vi "Open Method Front Panel.vi"(8 "error in (no error)":errorcluster, 10 "String":string, 11 "Execution UI In":refnum<class "Execution UI.lvclass">) -> (0 "error out":errorcluster, 3 "Execution UI Out":refnum<class "Execution UI.lvclass">)   [LabVIEW 2020, in "Execution UI.lvclass"]
uses:
  Execution UI.lvclass
  Execution UI.lvclass/Execution UI.ctl
  Helper Classes/Test Finder/Test Finder.lvclass
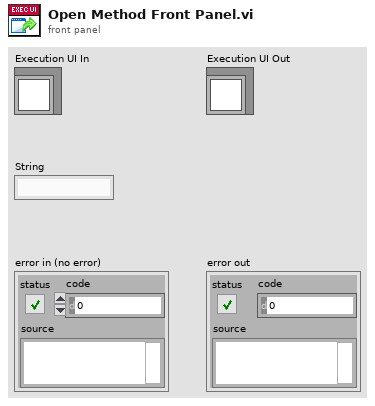
[diagram p1: front panel]
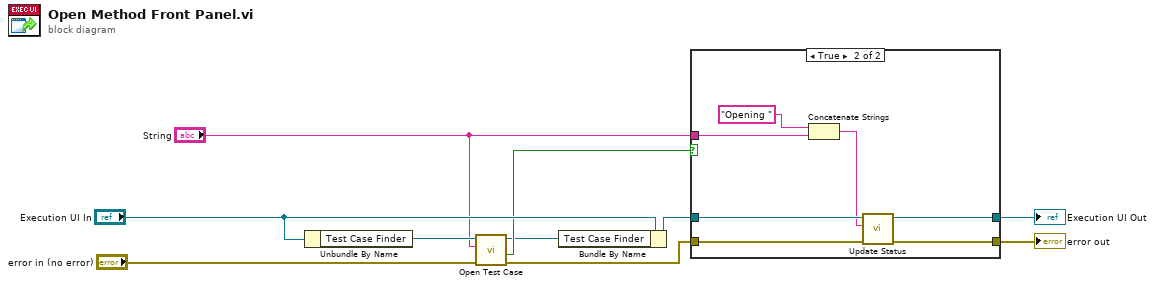
[diagram p0: block diagram]
diagram:
  n1 = Unbundle By Name("Execution UI In") -> ("Test Case Finder"=w10:refnum<class "Test Finder.lvclass">)
  n2 = call-dynamic "Open Test Case.vi"("error in (no error)"="error in (no error)", "Tag"="String", "Test Finder In"=w10) -> ("error out"=w6:errorcluster, "VI name valid?"=w7:bool, "Test Finder Out"=w1:refnum<class "Test Finder.lvclass">)  [unwired: 6 in]
  n3 = Bundle By Name(cluster="Execution UI In", "Test Case Finder"=w1) -> (w2:refnum<class "Execution UI.lvclass">)
  n4 = case shown="True" w7 {
    tunnel: w2 -> [w12 w19]
    tunnel: [w12 w18] -> w3
    tunnel: [w11 w17] -> w4
    tunnel: w6 -> [w11 w16]
    tunnel: "String" -> [_ w14]
    frame False {
    }
    frame True {
      n5 = Concatenate Strings("Opening " ("string"), w14) -> (w13:string)
      n6 = call "Update Status.vi"("error in (no error)"=w16, "Status"=w13, "Execution UI In"=w19) -> ("error out"=w17:errorcluster, "Execution UI Out"=w18:refnum<class "Execution UI.lvclass">)  [unwired: 7 in]
    }
  }
  "error out" <- w4
  "Execution UI Out" <- w3
